vi "Send Stage Abort Motion.vi"(7 "Message Priority (Normal)":T1=enum."Normal", 8 "error in (no error)":errorcluster, 11 "Message Enqueuer":refnum<class "Message Enqueuer.lvclass">) -> (0 "error out":errorcluster, 3 "Message Enqueuer out":refnum<class "Message Enqueuer.lvclass">)   [LabVIEW 2015, in "Application.lvlib" / "Stage Abort Motion Msg.lvclass"]
doc: "This VI sends the message to an actor."
uses:
  Stage Abort Motion Msg.lvclass
  <vilib>/ActorFramework/Message Enqueuer/Message Enqueuer.lvclass
  <vilib>/ActorFramework/Message Enqueuer/Message Priority.ctl
  <vilib>/ActorFramework/Message Enqueuer/Message Enqueuer.lvclass/Message Enqueuer.ctl
  <vilib>/ActorFramework/Message Priority Queue/Priority Enqueue.vi
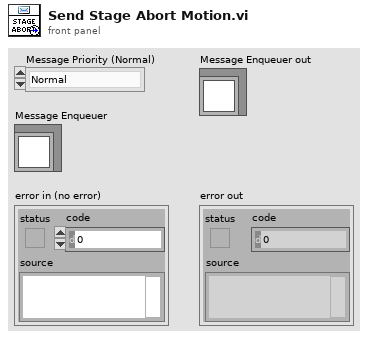
[diagram p1: front panel]
types:
  T1 = typedef "Actor Framework.lvlib/Message Enqueuer.lvclass/Message Priority.ctl" = enum16{"Low", "Normal", "High"}
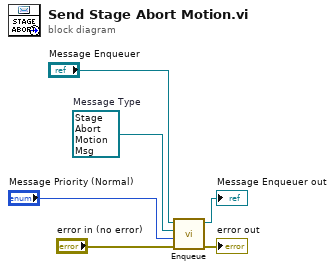
[diagram p0: block diagram]
diagram:
  w3 = refnum<class "Stage Abort Motion Msg.lvclass"> refnum  # Message Type
  n1 = call <vilib>:"Enqueue.vi"("error in (no error)"="error in (no error)", "Message Priority (Normal)"="Message Priority (Normal)", "Message"=w3, "Message Enqueuer in"="Message Enqueuer") -> ("error out"=→"error out":errorcluster, "Message Enqueuer out"=→"Message Enqueuer out":refnum<class "Message Enqueuer.lvclass">)  [unwired: 6 in]
